vi "NIIE_Selection_SetNewData.vi"(5 "#Active Layer":i32, 6 "Fire Ants Event? (T)":bool=TRUE, 7 "Error":errorcluster, 8 "Highlighted?":bool, 9 "All Layers":refnum<class "Layer.lvclass">[](array[class]), 10 "Data":T1={"Class"={"Ants"=refnum, "Layer"=refnum, "Templates"=refnum, "Icon"=refnum, "Glyph"=refnum, "Settings"=refnum, "Tools"=refnum}, "Ref"={"Add Layer"=refnum, "Remove Layer"=refnum, "Line Text"=[], "Body Text Spec"=refnum, "DNL_Font"=refnum, "glyph path str"=refnum, "templates path str"=refnum, "Arrow Up"=refnum, "Arrow Down"=refnum, "IE VI Ref"=refnum, "Glyphs tree"=refnum, "Templates tree"=refnum, "Layer Icon Text"=refnum, "Layer Template"=refnum, "Clipboard"=refnum, "BW icon in"=refnum, "Color icon in"=refnum, "Layer Clust"=refnum, "Body Text"=refnum, "DNL_Framework Templates"=refnum, "Search Templates"=refnum, "TextMarker"=refnum, "Tab Control"=refnum, "Search Glyphs"=refnum, "Line Color"=refnum, "DNL_Glyphs []"=refnum, "Fill Color"=refnum, "Tools"=refnum, "Glyphs tree"=refnum, "Icon"=refnum, "Preview"=refnum, "Ants"=refnum, "Terminals"=refnum, "menu reference"=refnum, "LayerNames"=[], "GlyphLoadAnimation"=refnum, "TemplateLoadAnimation"=refnum, "refreshGlyphs"=refnum, "refreshTemplates"=refnum}, "Support"={"AntsRect"={"left"=0, "top"=0, "right"=0, "bottom"=0}, "Mouse Move Coords"={"Horizontal"=0, "Vertical"=0}, "Mouse Down Coords"={"Horizontal"=0, "Vertical"=0}, "Temp Coord"={"Horizontal"=0, "Vertical"=0}, "Action"=enum."Default", "Edge Color"=4914962, "Fill Color"=16860, "Mouse Down?"=FALSE, "Draft Mode?"=FALSE, "Temp Icon"=bytes[3102], "CTRL Pressed"=FALSE, "Move Selection?"=FALSE, "AntsRect Orig"={"left"=0, "top"=0, "right"=0, "bottom"=0}, "Text"="", "TM Set?"=FALSE, "Mouse inside icon?"=FALSE, "Tool (old value)"=0, "Pencil Move Color"=0, "Swap Colors?"=FALSE, "Shift pressed?"=FALSE}}) -> (0 "Error Out":errorcluster, 1 "User Layers Out":refnum<class "Layer.lvclass">[](array[class]), 3 "Data Out":T1={"Class"={"Ants"=refnum, "Layer"=refnum, "Templates"=refnum, "Icon"=refnum, "Glyph"=refnum, "Settings"=refnum, "Tools"=refnum}, "Ref"={"Add Layer"=refnum, "Remove Layer"=refnum, "Line Text"=[], "Body Text Spec"=refnum, "DNL_Font"=refnum, "glyph path str"=refnum, "templates path str"=refnum, "Arrow Up"=refnum, "Arrow Down"=refnum, "IE VI Ref"=refnum, "Glyphs tree"=refnum, "Templates tree"=refnum, "Layer Icon Text"=refnum, "Layer Template"=refnum, "Clipboard"=refnum, "BW icon in"=refnum, "Color icon in"=refnum, "Layer Clust"=refnum, "Body Text"=refnum, "DNL_Framework Templates"=refnum, "Search Templates"=refnum, "TextMarker"=refnum, "Tab Control"=refnum, "Search Glyphs"=refnum, "Line Color"=refnum, "DNL_Glyphs []"=refnum, "Fill Color"=refnum, "Tools"=refnum, "Glyphs tree"=refnum, "Icon"=refnum, "Preview"=refnum, "Ants"=refnum, "Terminals"=refnum, "menu reference"=refnum, "LayerNames"=[], "GlyphLoadAnimation"=refnum, "TemplateLoadAnimation"=refnum, "refreshGlyphs"=refnum, "refreshTemplates"=refnum}, "Support"={"AntsRect"={"left"=0, "top"=0, "right"=0, "bottom"=0}, "Mouse Move Coords"={"Horizontal"=0, "Vertical"=0}, "Mouse Down Coords"={"Horizontal"=0, "Vertical"=0}, "Temp Coord"={"Horizontal"=0, "Vertical"=0}, "Action"=enum."Default", "Edge Color"=4914962, "Fill Color"=16860, "Mouse Down?"=FALSE, "Draft Mode?"=FALSE, "Temp Icon"=bytes[3102], "CTRL Pressed"=FALSE, "Move Selection?"=FALSE, "AntsRect Orig"={"left"=0, "top"=0, "right"=0, "bottom"=0}, "Text"="", "TM Set?"=FALSE, "Mouse inside icon?"=FALSE, "Tool (old value)"=0, "Pencil Move Color"=0, "Swap Colors?"=FALSE, "Shift pressed?"=FALSE}})   [LabVIEW 2021]
uses:
  vi.lib/LabVIEW Icon API/lv_icon/Classes/Layer/Layer.lvclass
  Controls/IE Data.ctl
  Class/Ants/Ants.lvclass
  Class/FakedArray/FakedArray.lvclass
  Class/Icon Library/Glyph.lvclass
  Class/Settings/Settings.lvclass
  Class/Tools/Tools Paint.lvclass
  vi.lib/LabVIEW Icon API/lv_icon/Classes/Icon/Icon.lvclass
  Controls/IE Classes.ctl
  Controls/References Cluster.ctl
  Controls/SupportClass.ctl
  <vilib>/Utility/miscctls.llb/LVPoint32TypeDef.ctl
  Controls/ENUM_SupportClass_Action.ctl
  vi.lib/LabVIEW Icon API/lv_icon/Controls/IEColor.ctl
  vi.lib/LabVIEW Icon API/lv_icon/Classes/Icon Framework/Icon Framework.lvclass
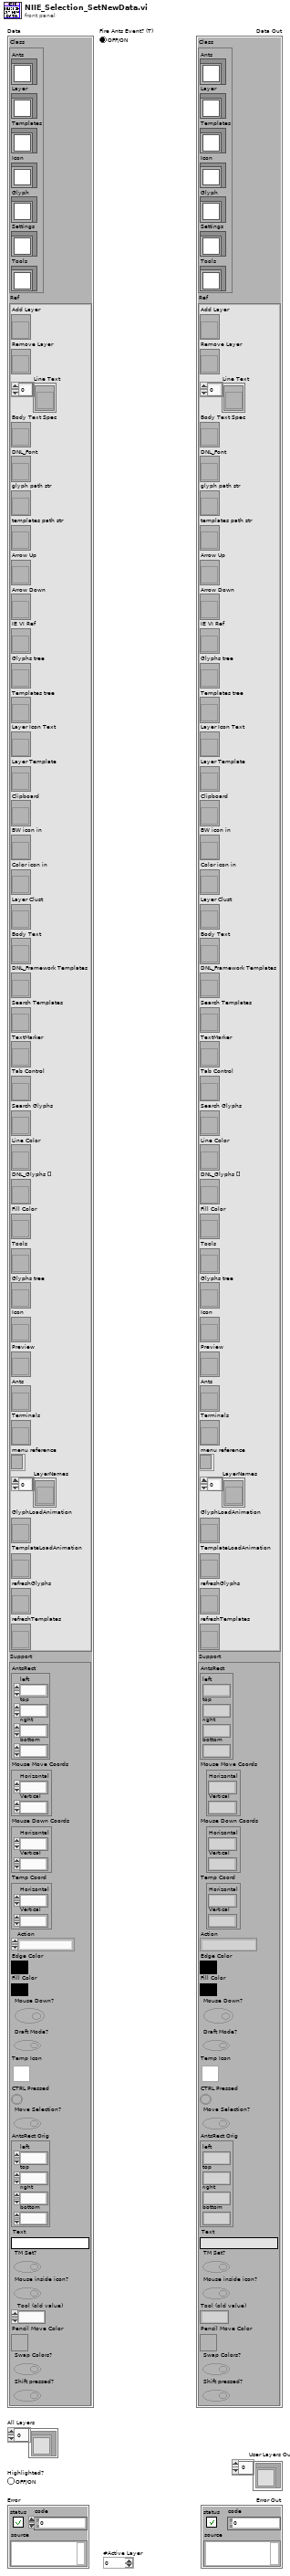
[diagram p1: front panel]
types:
  T1 = typedef "IE Data.ctl" = cluster{"Class":T2, "Ref":T3, "Support":T4}
  T2 = typedef "IE Classes.ctl" = cluster{"Ants":refnum<class "Ants.lvclass">, "Layer":refnum<class "FakedArray.lvclass">, "Templates":refnum<class "FakedArray.lvclass">, "Icon":refnum<class "Icon.lvclass">, "Glyph":refnum<class "Glyph.lvclass">, "Settings":refnum<class "Settings.lvclass">, "Tools":refnum<class "Tools Paint.lvclass">}
  T3 = typedef "References Cluster.ctl" = cluster{"Add Layer":refnum<vi>, "Remove Layer":refnum<vi>, "Line Text":refnum<vi>[], "Body Text Spec":refnum<vi>, "DNL_Font":refnum<vi>, "glyph path str":refnum<vi>, "templates path str":refnum<vi>, "Arrow Up":refnum<vi>, "Arrow Down":refnum<vi>, "IE VI Ref":refnum<vi>, "Glyphs tree":refnum<vi>, "Templates tree":refnum<vi>, "Layer Icon Text":refnum<vi>, "Layer Template":refnum<vi>, "Clipboard":refnum<vi>, "BW icon in":refnum<vi>, "Color icon in":refnum<vi>, "Layer Clust":refnum<vi>, "Body Text":refnum<vi>, "DNL_Framework Templates":refnum<vi>, "Search Templates":refnum<vi>, "TextMarker":refnum<vi>, "Tab Control":refnum<vi>, "Search Glyphs":refnum<vi>, "Line Color":refnum<vi>, "DNL_Glyphs []":refnum<vi>, "Fill Color":refnum<vi>, "Tools":refnum<vi>, "Glyphs tree":refnum<vi>, "Icon":refnum<vi>, "Preview":refnum<vi>, "Ants":refnum<vi>, "Terminals":refnum<vi>, "menu reference":refnum<k9>, "LayerNames":refnum<vi>[], "GlyphLoadAnimation":refnum<vi>, "TemplateLoadAnimation":refnum<vi>, "refreshGlyphs":refnum<vi>, "refreshTemplates":refnum<vi>}
  T4 = typedef "SupportClass.ctl" = cluster{"AntsRect":cluster{"left":i16, "top":i16, "right":i16, "bottom":i16}, "Mouse Move Coords":T5, "Mouse Down Coords":T5, "Temp Coord":T5, "Action":T6, "Edge Color":T7, "Fill Color":T7, "Mouse Down?":bool, "Draft Mode?":bool, "Temp Icon":picture, "CTRL Pressed":bool, "Move Selection?":bool, "AntsRect Orig":cluster{"left":i16, "top":i16, "right":i16, "bottom":i16}, "Text":string, "TM Set?":bool, "Mouse inside icon?":bool, "Tool (old value)":u32, "Pencil Move Color":u32, "Swap Colors?":bool, "Shift pressed?":bool}
  T5 = typedef "LVPoint32TypeDef.ctl" = cluster{"Horizontal":i32, "Vertical":i32}
  T6 = typedef "ENUM_SupportClass_Action.ctl" = enum16{"Default", "Move Selection", "Glyph Library", "Tool"}
  T7 = typedef "IEColor.ctl" = u32
  T8 = typedef "Cluster_Layer Data.ctl" = cluster{"LayerIcon":picture, "LayerName":string, "Opacity":u8, "Visibility?":bool}
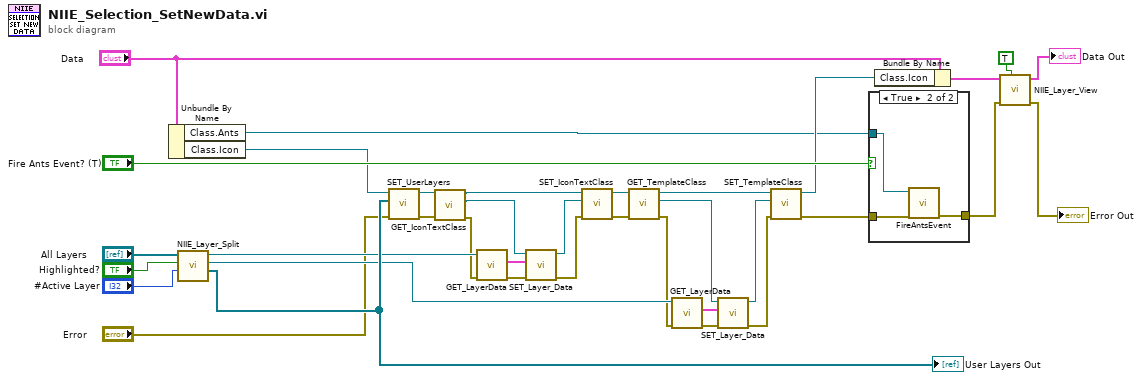
[diagram p0: block diagram]
diagram:
  n1 = Unbundle By Name("Data") -> ("Class.Ants"=w8:refnum<class "Ants.lvclass">, "Class.Icon"=w11:refnum<class "Icon.lvclass">)
  n2 = call "NIIE_Layer_Split.vi"("#Active Layer"="#Active Layer", "Is Highlighted?"="Highlighted?", "Layer out"="All Layers") -> ("User Layers"=w30:refnum<class "Layer.lvclass">[], "Template"=w26:refnum<class "Layer.lvclass">, "Icon Text"=w29:refnum<class "Layer.lvclass">)  [unwired: 6 out]
  "User Layers Out" <- w30
  n3 = call-dynamic "SET_UserLayers.vi"("error in (no error)"="Error", "Layers"=w30, "Icon.lvclass in"=w11) -> ("error out"=w17:errorcluster, "Icon.lvclass out"=w16:refnum<class "Icon.lvclass">)  [unwired: 7 in]
  n4 = call-dynamic "GET_IconTextClass.vi"("error in (no error)"=w17, "Icon.lvclass in"=w16) -> ("error out"=w13:errorcluster, "Icon Framework.lvclass"=w14:refnum<class "Icon Framework.lvclass">, "Icon.lvclass out"=w15:refnum<class "Icon.lvclass">)  [unwired: 7 out]
  n5 = call-dynamic "GET_LayerData.vi"("error in (no error)"=w13, "Layer.lvclass in"=w29) -> ("error out"=w22:errorcluster, "Data"=w28:T8)  [unwired: 8 out]
  n6 = call-dynamic "SET_Layer_Data.vi"("error in (no error)"=w22, "Data"=w28, "Layer.lvclass in"=w14) -> ("error out"=w21:errorcluster, "Layer.lvclass out"=w27:refnum<class "Icon Framework.lvclass">)  [unwired: 1 in, 6 out]
  n7 = call-dynamic "SET_IconTextClass.vi"("error in (no error)"=w21, "Icon Framework.lvclass"=w27, "Icon.lvclass in"=w15) -> ("error out"=w32:errorcluster, "Icon.lvclass out"=w33:refnum<class "Icon.lvclass">)  [unwired: 7 out]
  n8 = call-dynamic "GET_TemplateClass.vi"("error in (no error)"=w32, "Icon.lvclass in"=w33) -> ("error out"=w20:errorcluster, "Icon Framework.lvclass"=w24:refnum<class "Icon Framework.lvclass">, "Icon.lvclass out"=w34:refnum<class "Icon.lvclass">)  [unwired: 7 out]
  n9 = call-dynamic "GET_LayerData.vi"("error in (no error)"=w20, "Layer.lvclass in"=w26) -> ("error out"=w19:errorcluster, "Data"=w25:T8)  [unwired: 8 out]
  n10 = call-dynamic "SET_Layer_Data.vi"("error in (no error)"=w19, "Data"=w25, "Layer.lvclass in"=w24) -> ("error out"=w18:errorcluster, "Layer.lvclass out"=w23:refnum<class "Icon Framework.lvclass">)  [unwired: 1 in, 6 out]
  n11 = call-dynamic "SET_TemplateClass.vi"("error in (no error)"=w18, "Icon Framework.lvclass"=w23, "Icon.lvclass in"=w34) -> ("error out"=w1:errorcluster, "Icon.lvclass out"=w9:refnum<class "Icon.lvclass">)  [unwired: 7 out]
  n12 = case shown="True" "Fire Ants Event? (T)" {
    tunnel: [w37 w40] -> w3
    tunnel: w1 -> [w37 w39]
    tunnel: w8 -> [_ w38]
    frame False {
    }
    frame True {
      n13 = call "FireAntsEvent.vi"("error in (no error)"=w39, "Ants in"=w38) -> ("error out"=w40:errorcluster)  [unwired: 2 in, 7 out]
    }
  }
  n14 = Bundle By Name(cluster="Data", "Class.Icon"=w9) -> (w5:T1)
  n15 = call "NIIE_Layer_View.vi"("Add To Undo?"=TRUE ("Add to Undo?"), "Error"=w3, "Data"=w5) -> ("Error Out"=→"Error Out":errorcluster, "Data Out"=→"Data Out":T1)  [unwired: 1 in, 6 out]
